vi "Initialize_v0.vi"() -> ()   [LabVIEW 2021]
uses:
  <vilib>/Instr/_visa.llb/VISA Configure Serial Port (Instr).vi
  <vilib>/Utility/error.llb/Error Cluster From Error Code.vi
  <vilib>/ErrorRing/Error Ring.xnode
panel:
  out "return count":u32
  out "error IO":errorcluster
  in  "error in":errorcluster
  out "error out":errorcluster
  out "VISA resource name out":refnum<visa-resource-name>
  in  "VISA resource name":refnum<visa-resource-name>
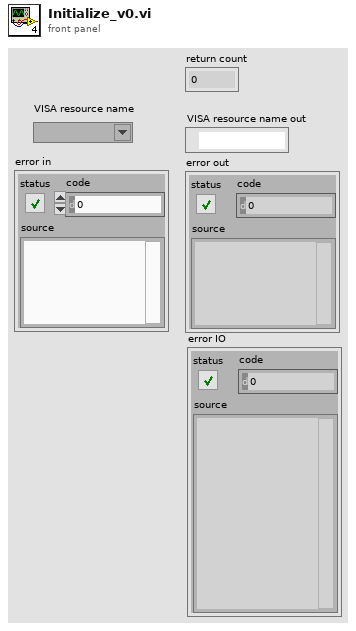
[diagram p1: front panel]
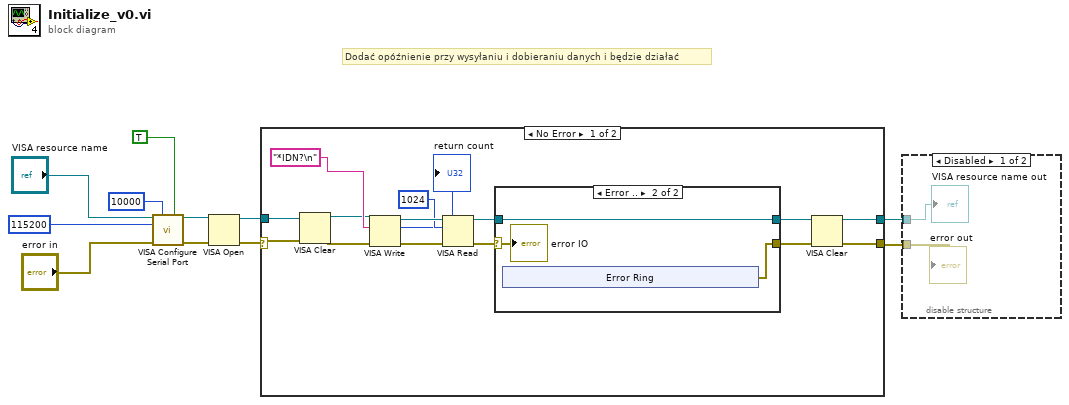
[diagram p0: block diagram]
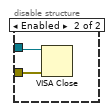
[diagram p2: hidden frame]
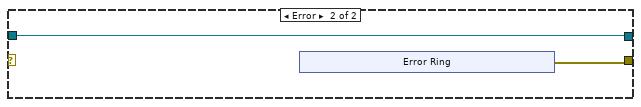
[diagram p4: hidden frame]
diagram:
  # "Dodać opóźnienie przy wysyłaniu i dobieraniu danych i będzie działać"
  n1 = call-poly "VISA Configure Serial Port"("VISA resource name"="VISA resource name", "timeout (10sec)"=u32 10000, "Enable Termination\nChar (T)"=TRUE ("Enable Termination\nChar (T)"), "baud rate (9600)"=u32 115200, "error in (no error)"="error in") -> ("VISA resource name out"=w8:refnum<visa-resource-name>, "error out"=w9:errorcluster)  [unwired: 9 in]
  n2 = VISA Open(error in (no error)=w9, VISA resource name=w8) -> (VISA resource name=w5:refnum<visa-resource-name>, error out=w7:errorcluster)  [unwired: 3 in]
  n3 = case shown="No Error" w7 {
    selector: w7 -> [w12 _]
    tunnel: [w20 w38] -> w6
    tunnel: w5 -> [w15 w37]
    tunnel: [w18 w37] -> w4
    frame No Error {
      n4 = VISA Clear(VISA resource name=w15, error in (no error)=w12) -> (VISA resource name out=w14:refnum<visa-resource-name>, error out=w13:errorcluster)
      n5 = VISA Write(VISA resource name=w14, write buffer="*IDN?\n", error in (no error)=w13) -> (VISA resource name out=w25:refnum<visa-resource-name>, return count=→"return count":u32, error out=w26:errorcluster)
      n6 = VISA Read(VISA resource name=w25, byte count=u32 1024, error in (no error)=w26) -> (VISA resource name out=w23:refnum<visa-resource-name>, error out=w24:errorcluster)  [unwired: 2 out]
      n7 = case shown="Error .." w24 {
        selector: w24 -> [w27 w29]
        tunnel: [w28 w30] -> w22
        tunnel: w23 -> [w28 w30]
        tunnel: [w27 w31] -> w21
        frame No Error {
        }
        frame Error {
          n8 = xnode "Error Ring"() -> ("error out"=w31:errorcluster)
          "error IO" <- w29
        }
      }
      n9 = VISA Clear(VISA resource name=w22, error in (no error)=w21) -> (VISA resource name out=w18:refnum<visa-resource-name>, error out=w20:errorcluster)
    }
    frame Error {
      n10 = xnode "Error Ring"() -> ("error out"=w38:errorcluster)
    }
  }
  n11 = disable-structure shown="Disabled" {
    disable-tunnel: w6 -> [w45 w47]
    disable-tunnel: w4 -> [w44 w46]
    frame Disabled {
      "VISA resource name out" <- w44
      "error out" <- w45
    }
    frame Enabled {
      n12 = VISA Close(VISA resource name=w46, error in (no error)=w47) -> ()  [unwired: 1 out]
    }
  }
